vi "Get camera FOVs.vi"(10 "Type":enum16{"Horizontal", "Vertical", "Diagonal"}(ring), 11 "Camera Type":T1) -> (1 "Camera view angles":dbl[](array[numeric])=[51.7, 49.4, 64.0, 52.0, 41.0], 3 "FOV":dbl=41.0)   [LabVIEW 2018]
doc: "Return the view angle for common FRC cameras. This is useful for calculating distances to objects in captured images."
uses:
  Camera Types.ctl
panel:
  in  "Camera view angles":dbl[][](array[numeric])=[[51.7, 49.4, 64.0, 49.2, 60.0], [32.0, 30.0, 38.0, 35.1, 35.0], [61.0, 58.0, 74.4, 61.0, 69.4]]
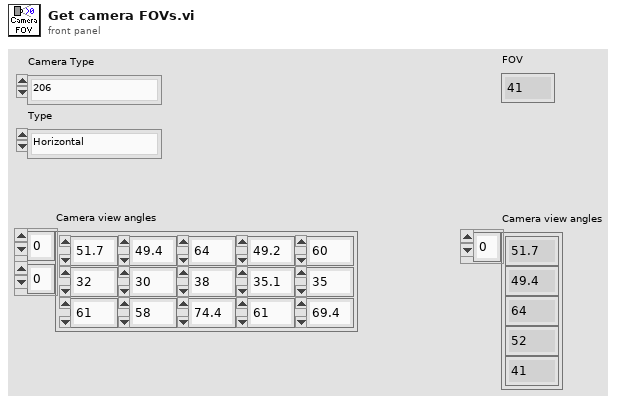
[diagram p1: front panel]
types:
  T1 = typedef "Camera Types.ctl" = enum16{"206", "1011", "1013", "MS HD3000 square", "MS HD3000 640x480"}
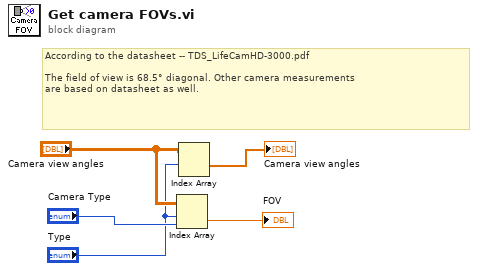
[diagram p0: block diagram]
diagram:
  # "According to the datasheet -- TDS_LifeCamHD-3000.pdf\n\nThe field of view is 68.5° diagonal. Other camera measurements\nare based on datasheet as well."
  n1 = Index Array(array="Camera view angles", index (row)="Type", index (col)="Camera Type") -> (element=→"FOV":dbl)
  n2 = Index Array(array="Camera view angles", index (row)="Type") -> (element=→"Camera view angles":dbl[])  [unwired: 1 in]
